vi "Network-Build TCP Message.vi"(0 "Code":i32=200, 5 "Command":string, 7 "Payload":string="{}") -> (8 "TCPMessage":T1)   [LabVIEW 2020]
uses:
  Typedefs/Network-TCP Message.ctl
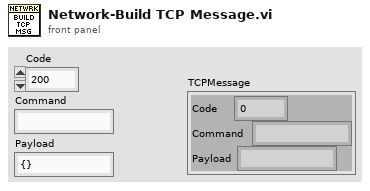
[diagram p1: front panel]
types:
  T1 = typedef "Network-TCP Message.ctl" = cluster{"Code":i32, "Command":string, "Payload":string}
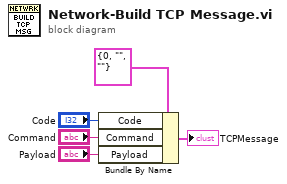
[diagram p0: block diagram]
diagram:
  n1 = Bundle By Name(cluster=T1 {"Code"=0, "Command"="", "Payload"=""} ("TCPMessage"), "Code"="Code", "Command"="Command", "Payload"="Payload") -> (→"TCPMessage":T1)
